vi "Get values from Variant.vi"(1 "Variant in":variant, 4 "Value in":i32) -> (5 "Value out":i32, 6 "Strings out":string[](array[string]), 7 "Disabled out":u8)   [LabVIEW 2018, in "Powermeter_library.lvlib"]
doc: "Converts a Variant returned by an ActiveX call into a list (string array) of items and the current index in that list. Also returns the disabled state (=2=disabled if item list is empty, otherwise =0=not disabled)"
uses:
  Powermeter_library.lvlib
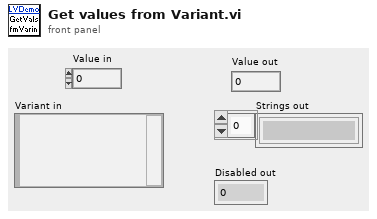
[diagram p1: front panel]
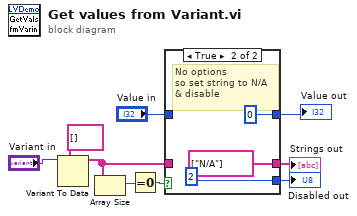
[diagram p0: block diagram]
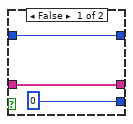
[diagram p2: hidden frame]
diagram:
  n1 = Variant To Data(type=string[] [], Variant="Variant in") -> (data=w6:string[])  [unwired: 1 in, 1 out]
  n2 = Array Size(array=w6) -> (size(s)=w5:i32)
  n3 = Equal To 0?(x=w5) -> (x = 0?=w9:bool)
  n4 = case shown="True" w9 {
    tunnel: w6 -> [w12 _]
    tunnel: [w12 string[] ["N/A"]] -> w7
    tunnel: [u8 0 ("f") u8 2 ("Disabled")] -> w8
    tunnel: "Value in" -> [w10 _]
    tunnel: [w10 0] -> w1
    frame False {
    }
    frame True {
      # "No options\nso set string to N/A\n& disable"
    }
  }
  "Disabled out" <- w8
  "Strings out" <- w7
  "Value out" <- w1
